vi "Get Card Map Hands and Profit-Loss.vi"(11 "Card Map In":T1(array[cluster])) -> (2 "Profit/Loss (BBs)":dbl, 3 "Total Hands":i32)   [LabVIEW 2021]
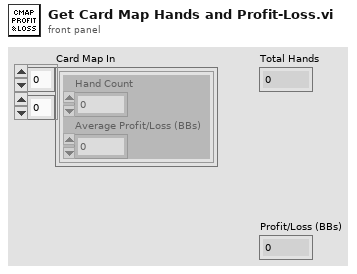
[diagram p1: front panel]
types:
  T1 = cluster{"Hand Count":u16, "Average Profit/Loss (BBs)":dbl}[][]
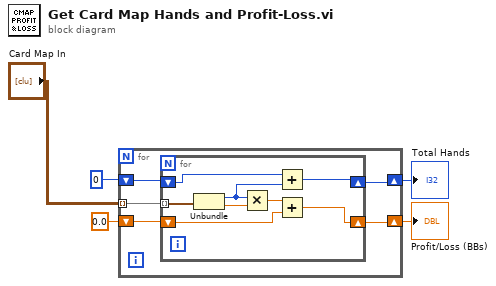
[diagram p0: block diagram]
diagram:
  n1 = for {
    tunnel: "Card Map In" -> [w10] mode=indexing
    shift-right: [w8] -> w3
    shift-left: 0.0 -> [w9]
    shift-right: [w6] -> w5
    shift-left: 0 -> [w7]
    n2 = for {
      tunnel: w10 -> [w18] mode=indexing
      shift-right: [w14] -> w8
      shift-left: w9 -> [w15]
      shift-right: [w11] -> w6
      shift-left: w7 -> [w13]
      n3 = Unbundle(w18) -> ("Hand Count"=w12:u16, "Average Profit/Loss (BBs)"=w17:dbl)
      n4 = Multiply(x=w12, y=w17) -> (x*y=w16:dbl)
      n5 = Add(x=w13, y=w12) -> (x+y=w11:i32)
      n6 = Add(x=w16, y=w15) -> (x+y=w14:dbl)
    }
  }
  "Total Hands" <- w5
  "Profit/Loss (BBs)" <- w3
